vi "Initialize.vi"(7 "Serial Configuration":T1={"Baud Rate"=115200, "Parity"=0, "Data Bits"=8, "Stop Bits"=10, "Flow Control"=0} {"Flow Control" items=["None", "XON/XOFF", "RTS/CTS", "XON/XOFF & RTS/CTS", "DTR/DSR", "XON/XOFF & DTR/DSR"]; "Stop Bits" items=["1.0"=10, "1.5"=15, "2.0"=20]; "Data Bits" items=["7"=7, "8"=8]; "Parity" items=["None", "Odd", "Even", "Mark", "Space"]; "Baud Rate" items=["300"=300, "600"=600, "1200"=1200, "2400"=2400, "4800"=4800, "9600"=9600, "19200"=19200]}, 8 "error in (no error)":errorcluster, 10 "ID Query (True)":bool=TRUE, 11 "VISA resource name":refnum<visa-resource-name>) -> (0 "error out":errorcluster, 3 "VISA resource name out":refnum<visa-resource-name>)   [LabVIEW 2012, in "YOST 3 Space.lvlib"]
uses:
  YOST 3 Space.lvlib
  Motors/Roboteq/Roboteq.lvlib
panel:
  out "read buffer":string
  out "error out 2":errorcluster
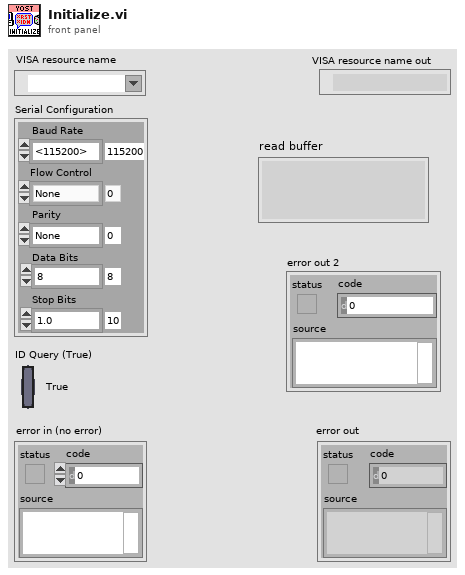
[diagram p1: front panel]
types:
  T1 = cluster{"Baud Rate":u32, "Parity":u16, "Data Bits":u16, "Stop Bits":u16, "Flow Control":u16}
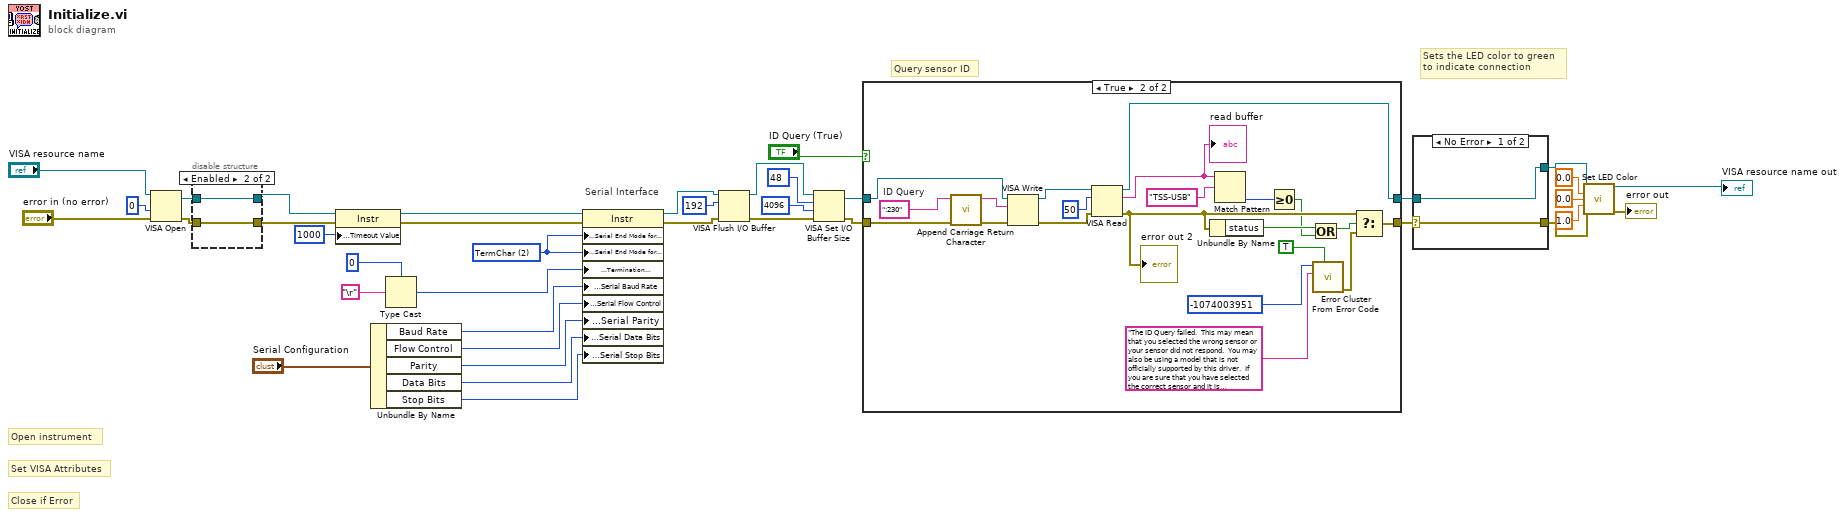
[diagram p0: block diagram]
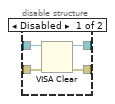
[diagram p2: hidden frame]
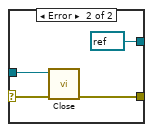
[diagram p3: hidden frame]
diagram:
  w15 = u16 2 items=["None", "LastBit", "TermChar"] ("Serial Settings:Serial End Mode for Reads")
  # "Sets the LED color to green to indicate connection"
  # "Serial Interface"
  # "Set VISA Attributes"
  # "Close if Error"
  # "Query sensor ID"
  # "Open instrument"
  n1 = VISA Open(access mode=u32 0, error in (no error)="error in (no error)", VISA resource name="VISA resource name") -> (VISA resource name=w30:refnum<visa-resource-name>, error out=w29:errorcluster)  [unwired: 2 in]
  n2 = disable-structure shown="Enabled" {
    disable-tunnel: w30 -> [w43 w45]
    disable-tunnel: w29 -> [w42 w44]
    disable-tunnel: [w41 w45] -> w28
    disable-tunnel: [w40 w44] -> w27
    frame Disabled {
      n3 = VISA Clear(VISA resource name=w43, error in (no error)=w42) -> (VISA resource name out=w41:refnum<visa-resource-name>, error out=w40:errorcluster)
    }
    frame Enabled {
    }
  }
  n4 = property class="Instr"(reference=w28, error in=w27, "General Settings:Timeout Value"=u32 1000) -> (reference out=w33:refnum<visa-resource-name>, error out=w32:errorcluster)
  n5 = Unbundle By Name("Serial Configuration") -> ("Baud Rate"=w13:u32, "Flow Control"=w9:u16, "Parity"=w11:u16, "Data Bits"=w12:u16, "Stop Bits"=w8:u16)
  n6 = Type Cast(type=u8 0, x="\r") -> (*(type *) &x=w14:u8)
  n7 = property class="Instr"(reference=w33, error in=w32, "Serial Settings:Serial End Mode for Reads"=w15, "Serial Settings:Serial End Mode for Writes"=w15, "Message Based Settings:Termination Character"=w14, "Serial Settings:Serial Baud Rate"=w13, "Serial Settings:Serial Flow Control"=w9, "Serial Settings:Serial Parity"=w11, "Serial Settings:Serial Data Bits"=w12, "Serial Settings:Serial Stop Bits"=w8) -> (reference out=w21:refnum<visa-resource-name>, error out=w23:errorcluster)
  n8 = VISA Flush I/O Buffer(VISA resource name=w21, mask (16)=u16 192, error in (no error)=w23) -> (VISA resource name out=w24:refnum<visa-resource-name>, error out=w22:errorcluster)
  n9 = VISA Set I/O Buffer Size(VISA resource name=w24, mask (16)=u16 48, size (4096)=u32 4096 ("size (0)"), error in (no error)=w22) -> (VISA resource name out=w35:refnum<visa-resource-name>, error out=w34:errorcluster)
  n10 = case shown="True" "ID Query (True)" {
    tunnel: [w46 w68] -> w25
    tunnel: [w47 w66] -> w26
    tunnel: w35 -> [w47 w67]
    tunnel: w34 -> [w46 w51]
    frame False {
    }
    frame True {
      w48 = ":230"  # ID Query
      n11 = call "Append Carriage Return Character.vi"("error in (no error)"=w51, "Command"=w48) -> ("error out"=w50:errorcluster, "Command Out"=w49:string)  [unwired: 8 in]
      n12 = VISA Write(VISA resource name=w67, write buffer=w49, error in (no error)=w50) -> (VISA resource name out=w64:refnum<visa-resource-name>, error out=w63:errorcluster)  [unwired: 1 out]
      n13 = VISA Read(VISA resource name=w64, byte count=u32 50, error in (no error)=w63) -> (VISA resource name out=w66:refnum<visa-resource-name>, read buffer=w65:string, error out=w55:errorcluster)  [unwired: 1 out]
      "read buffer" <- w65
      "error out 2" <- w55
      n14 = Unbundle By Name(w55) -> ("status"=w54:bool)
      n15 = Match Pattern(string=w65, regular expression="TSS-USB") -> (offset past match=w56:i32)  [unwired: 1 in, 3 out]
      n16 = Greater Or Equal To 0?(x=w56) -> (x >= 0?=w53:bool)
      n17 = Or(x=w54, y=w53) -> (x .or. y?=w52:bool)
      n18 = call <vilib>:"Error Cluster From Error Code.vi"("show call chain? (False)"=TRUE, "error message (\"\")"="The ID Query failed.  This may mean that you selected the wrong sensor or your sensor did not respond.  You may also be using a model that is not officially supported by this driver.  If you are sure that you have selected the correct sensor and it is responding, try disabling the ID Query." ("Source (VI Name)"), "error code (0)"=-1074003951 ("Code")) -> ("error out"=w60:errorcluster)  [unwired: 6 in]
      n19 = Select(t=w55, s=w52, f=w60) -> (s? t:f=w68:errorcluster)
    }
  }
  n20 = case shown="No Error" w25 {
    selector: w25 -> [w69 w72]
    tunnel: w26 -> [w70 w73]
    tunnel: [w70 refnum<visa-resource-name> refnum ("VISA resource name out")] -> w3
    tunnel: [w69 w74] -> w2
    frame No Error {
    }
    frame Error {
      n21 = call "Close.vi"("error in (no error)"=w72, "VISA resource name"=w73) -> ("error out"=w74:errorcluster)  [unwired: 9 in]
    }
  }
  n22 = call "Set LED Color.vi"("Session In"=w3, "Red"=0.0, "Blue"=0.0, "Green"=1.0, "error in"=w2) -> ("Session Out"=→"VISA resource name out":refnum<visa-resource-name>, "error out"=→"error out":errorcluster)  [unwired: 9 in]
